vi "init.vi"(8 "error in":errorcluster, 10 "TBM module configuration in":refnum<class "TBM module configuration.lvclass">, 11 "EIP Tags Runtime in":refnum<class "EIP Tags Runtime.lvclass">) -> (0 "error out":errorcluster, 1 "data allocations":T1, 2 "execution settings":T4, 3 "EIP Tags Runtime out":refnum<class "EIP Tags Runtime.lvclass">)   [LabVIEW 2013, in "EIP Tags Runtime.lvclass"]
doc: "Provides an interface for initializing a module at runtime. While this interface performs no operations, a child should provide an override which may open any necessary references or sessions, allocate necessary memory, and perform any final configuration validataion before providing the full configuration <b>execution data</b> to the calling process."
uses:
  EIP Tags Runtime.lvclass
  <vilib>/NI/Tag Bus Module Framework/channel/TBM channel.lvclass
  <vilib>/NI/Tag Bus Module Framework/runtime/TBM module execution interface.lvclass
  configuration/EIP Tags Configuration.lvclass
  <vilib>/NI/Tag Bus Module Framework/module configuration/TBM module configuration.lvclass
  <vilib>/NI/Tag Bus Module Framework/runtime/execution settings.ctl
  <vilib>/NI/Tag Bus Module Framework/channel/data tables.ctl
  <vilib>/NI/Tag Bus/dictionary/data dictionary.lvclass
  <vilib>/NI/Tag Bus/dictionary table pair.ctl
  <vilib>/NI/Tag Bus/tag bus.lvlib
  <vilib>/NI/Tag Bus/table/data table.ctl
  <vilib>/NI/Tag Bus/table/data table.lvlib
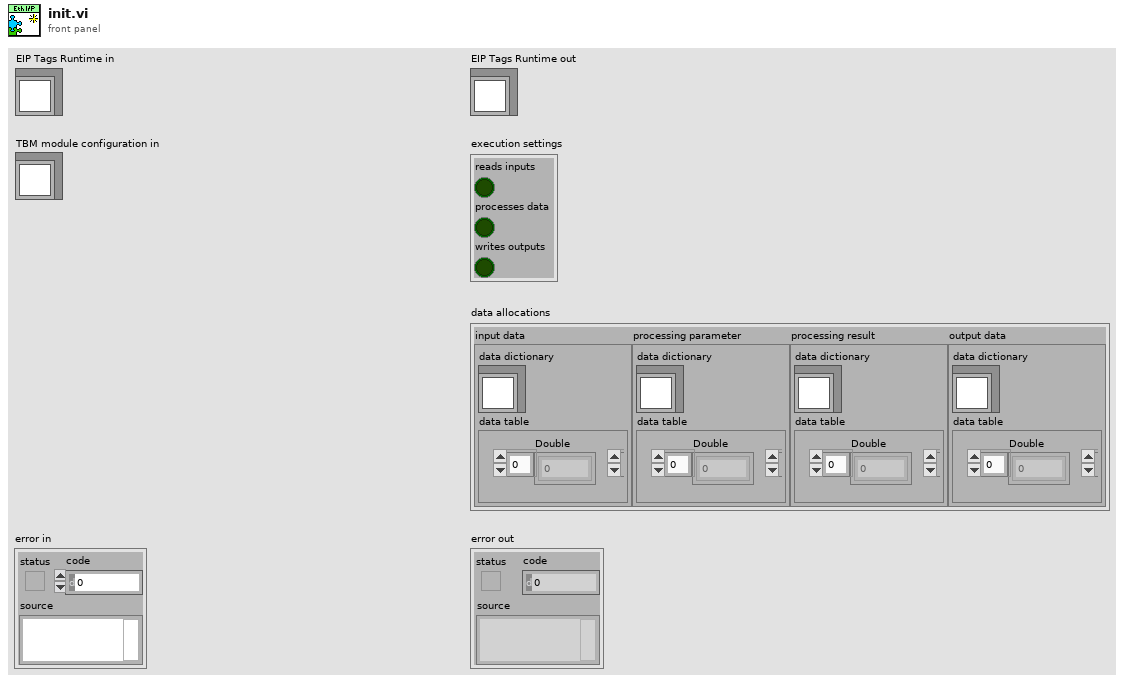
[diagram p1: front panel]
types:
  T1 = typedef "TBM channel.lvclass/data tables.ctl" = cluster{"input data":T2, "processing parameter":T2, "processing result":T2, "output data":T2}
  T2 = typedef "tag bus.lvlib/dictionary table pair.ctl" = cluster{"data dictionary":refnum<class "data dictionary.lvclass">, "data table":T3}
  T3 = typedef "tag bus.lvlib/data table.lvlib/data table.ctl" = cluster{"Double":dbl[], "Single":sgl[], "I64":i64[], "I32":i32[], "I16":i16[], "I8":i8[], "U64":u64[], "U32":u32[], "U16":u16[], "U8":u8[], "Boolean":bool[], "String":string[], "Array of Double":cluster{"DBL Array":dbl[]}[], "Array of Single":cluster{"SGL Array":sgl[]}[], "Array of I64":cluster{"I64 Array":i64[]}[], "Array of I32":cluster{"I32 Array":i32[]}[], "Array of I16":cluster{"I16 Array":i16[]}[], "Array of I8":cluster{"I8 Array":i8[]}[], "Array of U64":cluster{"U64 Array":u64[]}[], "Array of U32":cluster{"U32 Array":u32[]}[], "Array of U16":cluster{"U16 Array":u16[]}[], "Array of U8":cluster{"U8 Array":u8[]}[], "Array of Boolean":cluster{"Boolean Array":bool[]}[], "Array of String":cluster{"String Array":string[]}[]}
  T4 = typedef "TBM module execution interface.lvclass/execution settings.ctl" = cluster{"reads inputs":bool, "processes data":bool, "writes outputs":bool}
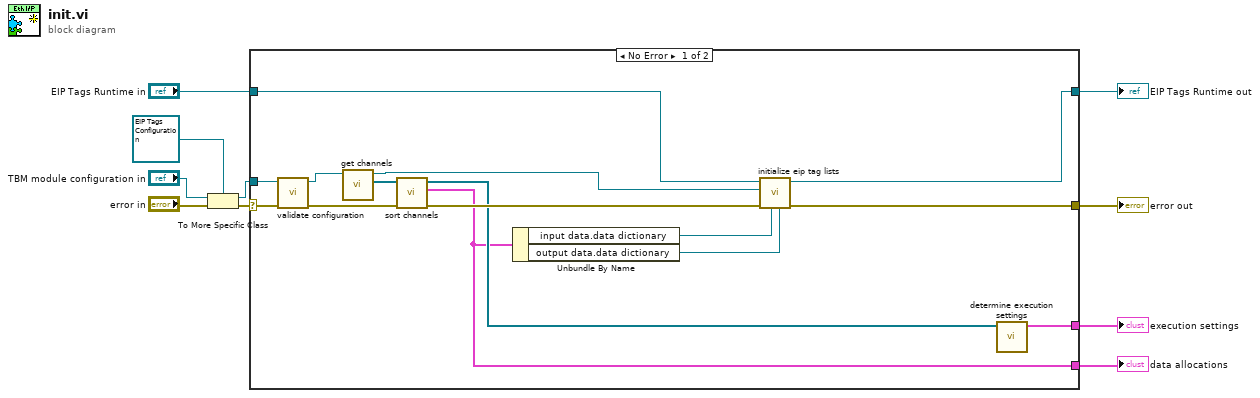
[diagram p0: block diagram]
diagram:
  n1 = To More Specific Class(target class=refnum<class "EIP Tags Configuration.lvclass"> refnum ("Synchronous module configuration"), reference="TBM module configuration in", error in="error in") -> (specific class reference=w9:refnum<class "EIP Tags Configuration.lvclass">, error out=w10:errorcluster)
  n2 = case shown="No Error" w10 {
    selector: w10 -> [w20 w26]
    tunnel: w9 -> [w19 _]
    tunnel: "EIP Tags Runtime in" -> [w25 w27]
    tunnel: [w15 w27] -> w4
    tunnel: [w16 w26] -> w3
    tunnel: [w13 _] -> w1
    tunnel: [w23 _] -> w2
    frame No Error {
      n3 = call-dynamic "validate configuration.vi"("error in"=w20, "EthernetIP configuration in"=w19) -> ("error out"=w21:errorcluster, "EthernetIP configuration out"=w18:refnum<class "EIP Tags Configuration.lvclass">)  [unwired: 8 in]
      n4 = call-dynamic "get channels.vi"("EthernetIP configuration in"=w18) -> ("channels"=w17:refnum<class "TBM channel.lvclass">[], "EthernetIP configuration out"=w14:refnum<class "EIP Tags Configuration.lvclass">)  [unwired: 9 in]
      n5 = call <vilib>:"sort channels.vi"("error in"=w21, "channels in"=w17) -> ("error out"=w24:errorcluster, "data allocations"=w13:T1, "channels out"=w22:refnum<class "TBM channel.lvclass">[])  [unwired: 7 in]
      n6 = Unbundle By Name(w13) -> ("input data.data dictionary"=w11:refnum<class "data dictionary.lvclass">, "output data.data dictionary"=w12:refnum<class "data dictionary.lvclass">)
      n7 = call "initialize eip tag lists.vi"("output dictionary"=w12, "input dictionary"=w11, "error in"=w24, "EthernetIP configuration in"=w14, "EthernetIP runtime in"=w25) -> ("error out"=w16:errorcluster, "EthernetIP runtime out"=w15:refnum<class "EIP Tags Runtime.lvclass">)  [unwired: 5 in]
      n8 = call <vilib>:"determine execution settings.vi"("channels"=w22) -> ("execution settings"=w23:T4)  [unwired: 10 in]
    }
    frame Error {
    }
  }
  "error out" <- w3
  "EIP Tags Runtime out" <- w4
  "execution settings" <- w2
  "data allocations" <- w1
